vi "NanotecSMCPD.reset.vi"(0 "i ref in":refnum<vi>, 3 "ms timeout (10000)":i32=10000, 5 "error in (no error)":errorcluster) -> (14 "i ref out":refnum<vi>, 17 "timed out":bool, 19 "error out":errorcluster)   [LabVIEW 2014, in "NanotecSMCPD.lvlib"]
doc: "Resets all axes."
uses:
  NanotecSMCPD.lvlib
  CSCore/CSSystem/CoreDefs/CoreDefs.error_type.ctl
  CSCore/CSSystem/CoreDefs/CoreDefs.error_severity.ctl
  CSCore/CSApplicationBaseClasses/MotorBase/MotorBase.lvlib
  CSCore/CSSystem/CoreLib/CoreLib.lvlib
  CSCore/CSApplicationBaseClasses/DeviceBase/DeviceBase.lvlib
  CSlibraries/UtilityLib/UtilityLib.lvlib
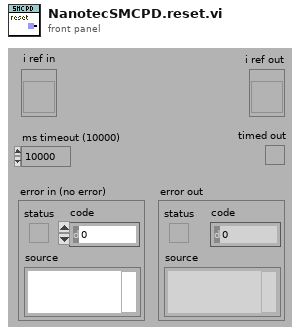
[diagram p1: front panel]
types:
  T1 = typedef "CoreDefs.error_severity.ctl" = enum16{"undefined", "information", "warning", "error", "fatal"}
  T2 = typedef "CoreDefs.error_type.ctl" = enum16{"no error", "can't load process", "can't unload process", "process does not exist", "can't install process", "can't remove process", "unknown function", "time out", "can't execute function", "duplicate queue name", "super not found", "caller queue invalid", "can't ping process", "unknown error", "VISA Error", "VISA timeout", "GPIB timeout", "GPIB error", "communication error", "data type mismatch", "can't read data from OPC server", "can't write data to OPC server", "OET error", "function not implemented", "process already exists", "invalid Shared Variable name", "error writing Shared Variable", "error reading Shared Variable", "invalid client name", "corrupt database", "unknown class", "call not authorized", "parameter out of range", "OET timeout: can't get data to modify", "invalid queue name", "requested operation incompatible with current state", "event undefined", "event disabled", "state undefined", "caller is not a friend", "EventBuilder: bad eventID", "EventBuilder: no DAQ devices", "a thread must not stop itself", "UNUSED ELEMENT4", "DiscArchiver: eventData incomplete", "DiscArchiver: eventData does not belong to run", "DiscArchiver: can't open file", "DiscArchiver: can't write to file", "DiscArchiver: available disc space low", "can't acquire semaphore", "error reading data from database", "notifier object is not existing", "can't register process", "can't unregister process", "illegal event type", "object disabled", "object already exists", "can't change state", "Instrument not found", "no connection to remote node", "invalid reference", "N/A", "UNUSED ELEMENT 1", "element not found", "illegal TCP/IP connection detected", "object does not exist", "invalid access ID", "unknown CS system", "invalid privilige", "unsupported data type", "unsupported server type", "IO server already exists", "Shared Variable already exists"}
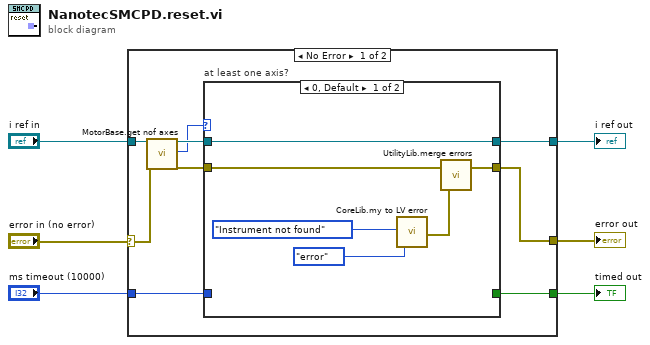
[diagram p0: block diagram]
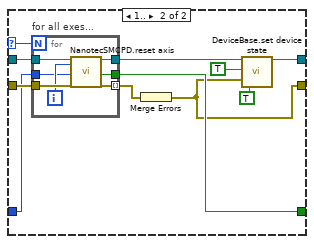
[diagram p2: hidden frame]
diagram:
  n1 = case shown="No Error" "error in (no error)" {
    selector: "error in (no error)" -> [w13 w40]
    tunnel: "i ref in" -> [w15 w41]
    tunnel: [w9 w41] -> w5
    tunnel: [w8 w40] -> w4
    tunnel: "ms timeout (10000)" -> [w12 _]
    tunnel: [w7 _] -> w1
    frame No Error {
      n2 = call "MotorBase.get nof axes.vi"("i ref in"=w15, "error in (no error)"=w13) -> ("i ref out"=w14:refnum<vi>, "nOfAxis"=w10:i32, "error out"=w11:errorcluster)  [unwired: 15 in]
      n3 = case "at least one axis?" shown="0, Default" w10 {
        selector: w10 -> [_ w32]
        tunnel: w14 -> [w21 w31]
        tunnel: w12 -> [_ w29]
        tunnel: w11 -> [w16 w30]
        tunnel: [w21 w26] -> w9
        tunnel: [w17 w22] -> w8
        tunnel: [_ w28] -> w7
        frame 0, Default {
          n4 = call "CoreLib.my to LV error.vi"("ErrorTypes"=CoreDefs.error_type."Instrument not found", "severityLevel"=CoreDefs.error_severity."error") -> ("myErrorCluster"=w18:errorcluster)  [unwired: 16 in, 1 out]
          n5 = call "UtilityLib.merge errors.vi"("error2 (no error)"=w18, "error1 (no error)"=w16) -> ("error out"=w17:errorcluster)
        }
        frame 1.. {
          n6 = for "for all exes..." {
            N: w32 -> [_]
            tunnel: w31 -> [w39]
            tunnel: [w35] -> w27
            tunnel: w29 -> [w36]
            tunnel: [w33] -> w28
            tunnel: w30 -> [w38]
            tunnel: [w34] -> w23 mode=indexing
            i -> [w37]
            n7 = call "NanotecSMCPD.reset axis.vi"("i ref in"=w39, "axis"=w37, "ms timeout (10000)"=w36, "error in (no error)"=w38) -> ("i ref out"=w35:refnum<vi>, "timed out"=w33:bool, "error out"=w34:errorcluster)  [unwired: 13 in]
          }
          n8 = Merge Errors(w23) -> (w22:errorcluster)
          n9 = call "DeviceBase.set device state.vi"("i ref in"=w27, "implicit"=TRUE, "device error"=w22, "mayResetError (FALSE)"=TRUE) -> ("i ref out"=w26:refnum<vi>)  [unwired: 13 in, 2 out]
        }
      }
    }
    frame Error {
    }
  }
  "error out" <- w4
  "i ref out" <- w5
  "timed out" <- w1
